vi "read work position.vi"(8 "error in (no error)":errorcluster caption="错误输入（无错误）") -> (0 "error out":errorcluster caption="错误输出", 3 "Work Position":i32[](array[numeric]))   [LabVIEW 2015]
uses:
  <vilib>/Utility/config.llb/Read Key (I32).vi
  <vilib>/Utility/config.llb/NI_LVConfig.lvlib
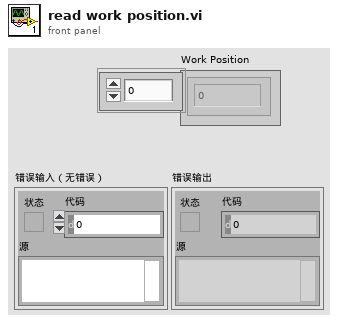
[diagram p1: front panel]
types:
  T1 = typedef "NI_LVConfig.lvlib/Config Data RefNum.ctl" = refnum<k1>
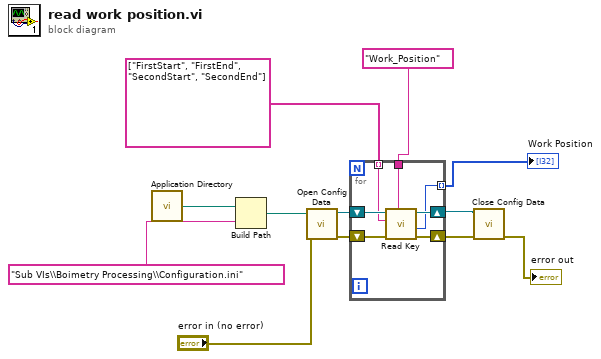
[diagram p0: block diagram]
diagram:
  n1 = call <vilib>:"Application Directory.vi"() -> ("Application Directory"=w10:path)
  n2 = Build Path(base path=w10, name or relative path="Sub VIs\\Boimetry Processing\\Configuration.ini" ("名称或相对路径")) -> (appended path=w8:path)
  n3 = call <vilib>:"Open Config Data.vi"("error in (no error)"="error in (no error)", "configuration file path"=w8) -> ("error out"=w12:errorcluster, "refnum"=w11:T1)  [unwired: 7 in, 1 out]
  n4 = for {
    tunnel: "Work_Position" ("section") -> [w17]
    shift-right: [w16] -> w6
    shift-left: w11 -> [w19]
    shift-right: [w15] -> w7
    shift-left: w12 -> [w18]
    tunnel: string[] ["FirstStart", "FirstEnd", "SecondStart", "SecondEnd"] -> [w13] mode=indexing
    tunnel: [w14] -> w3 mode=indexing
    n5 = call-poly <vilib>:"Read Key.vi"("section"=w17, "error in (no error)"=w18, "key"=w13, "refnum"=w19) -> ("error out"=w15:errorcluster, "value"=w14:i32, "refnum out"=w16:T1)  [unwired: 4 in, 1 out]
  }
  "Work Position" <- w3
  n6 = call <vilib>:"Close Config Data.vi"("error in (no error)"=w7, "refnum"=w6) -> ("error out"=→"error out":errorcluster)  [unwired: 8 in, 1 out]
